vi "Cluster_Analysis.vi"(2 "Shift In":T1[](array[typedef])) -> (0 "Shift Out":T1[](array[typedef]))   [LabVIEW 2014]
uses:
  Controls/Shift_Cluster.ctl
  Controls/XY_Plot_Cluster.ctl
  Controls/Inst_type.ctl
  Globals/Meas_global.vi
  Globals/LDA_meas_global_1.vi
  Globals/LDA_meas_global_2.vi
  <vilib>/Analysis/NI_AALBase.lvlib
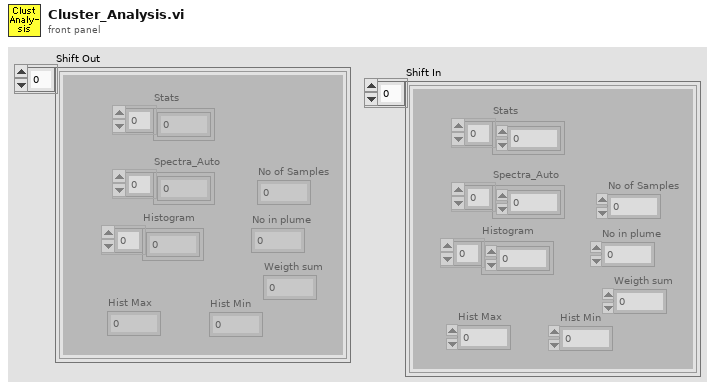
[diagram p1: front panel]
types:
  T1 = typedef "Shift_Cluster.ctl" = cluster{"Stats":dbl[], "Spectra_Auto":dbl[], "Histogram":dbl[], "Hist Max":dbl, "Hist Min":dbl, "No of Samples":i32, "No in plume":i32, "Weigth sum":dbl}
  T2 = typedef "Analysis_info_cluster.ctl" = cluster{"Colour":u32, "Inst type":T3, "Inst name":string, "Symbol":string, "Code name":string, "Extra Info":string, "Inst Array":T4, "Extra Titles":string[], "Extra Values":string[], "U":dbl, "u^2":dbl, "u^3":dbl, "u^4":dbl, "Skew_u":dbl, "Kurt_u":dbl, "Sd Error in Mean":dbl, "% u'/U":dbl, "X":dbl, "Y":dbl, "Z":dbl, "Timescale integral to 25%":dbl, "Sd Error in Variance":dbl, "Calib File":path, "Calib Constants":dbl[], "Output Position":bool, "Full Stats":bool, "Av Sampling Rate":dbl, "Av No of Samples":dbl, "Total Meas Time (s)":dbl, "ADAM Ch Name":string}
  T3 = typedef "Inst_type.ctl" = enum16{"Propeller anemometer", "Raw voltage", "Pressure Transducer", "Pitot-static tube", "Preston tube", "Hot wire", "Cross wire 1", "Cross wire 2", "Generic Linear", "Generic Polynomial", "Generic BackPoly", "Fast FID", "Thermocouple", "Cold wire", "Pulsed Wire", "LDA Vel", "LDA Tran time", "LDA Arr time", "Microphone"}
  T4 = typedef "Instrument_Array.ctl" = enum16{"PWA", "LDA", "Analogue"}
  T5 = typedef "Time_Trace_Cluster.ctl" = cluster{"Weighting":dbl[], "Time (s)":dbl[], "Voltage":dbl[], "Eng Values":dbl[]}
  T6 = typedef "XY_Plot_Cluster.ctl" = cluster{"First Name":string, "Second Name":string, "X axis name":string, "Y axis name":string, "X array":dbl[], "Y array":dbl[]}
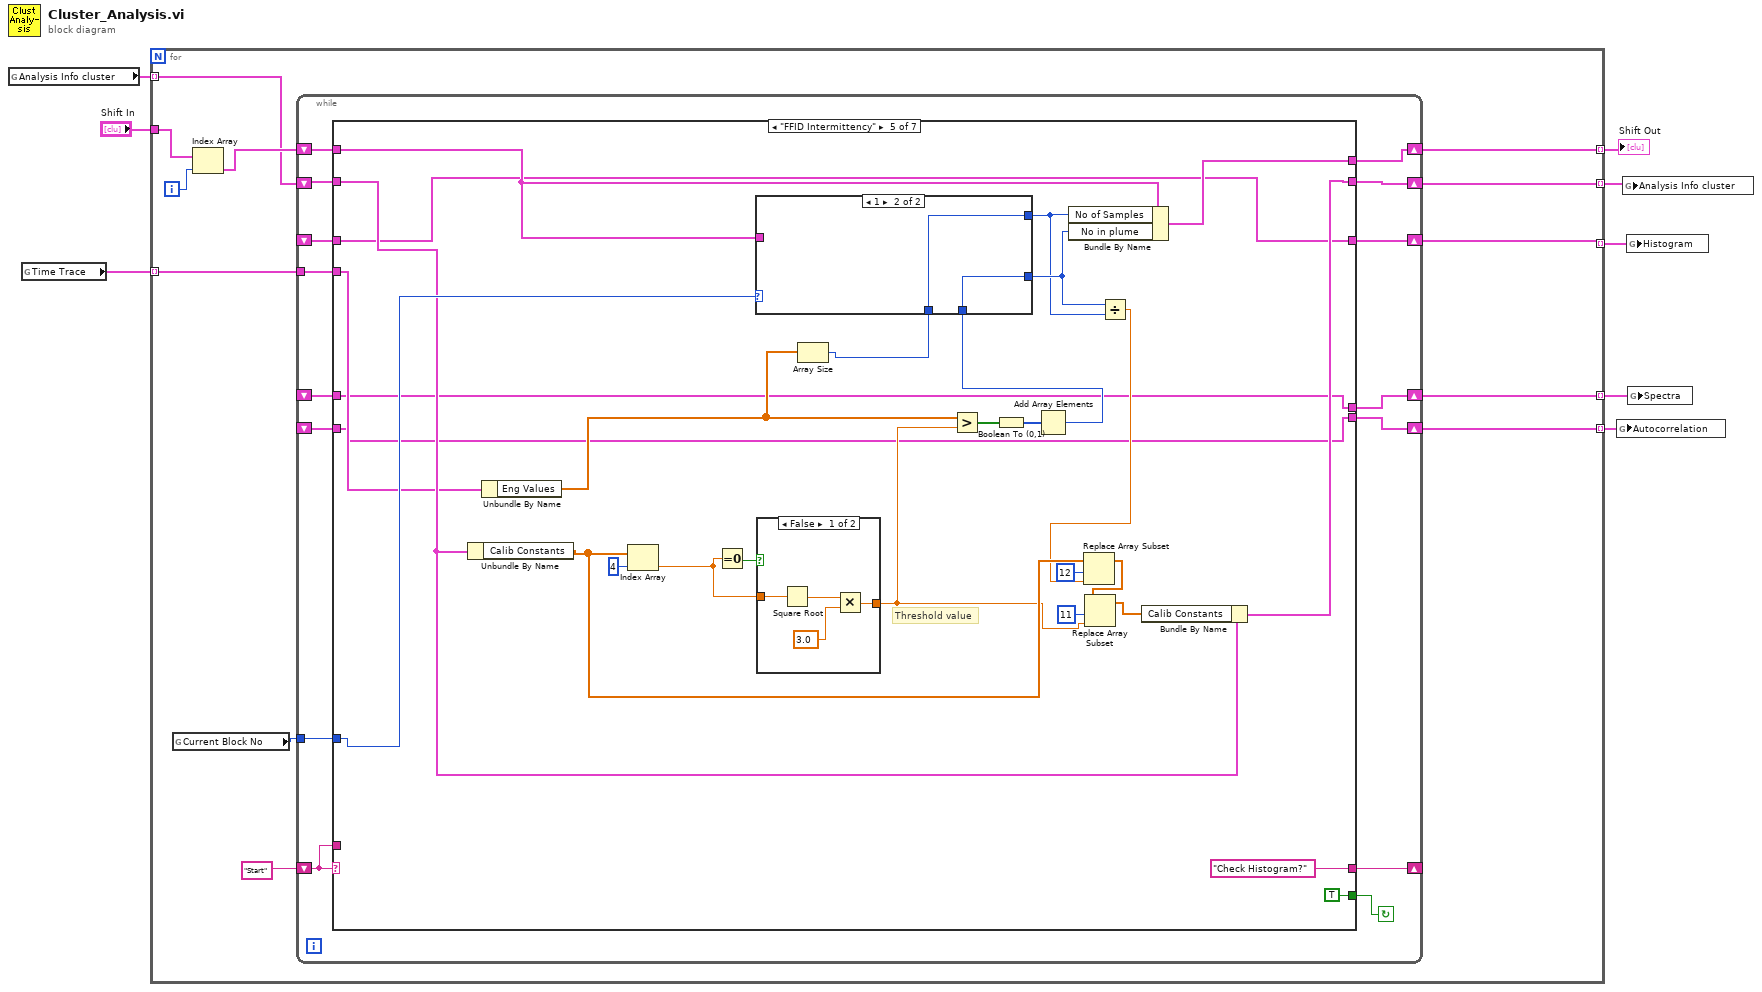
[diagram p0: block diagram]
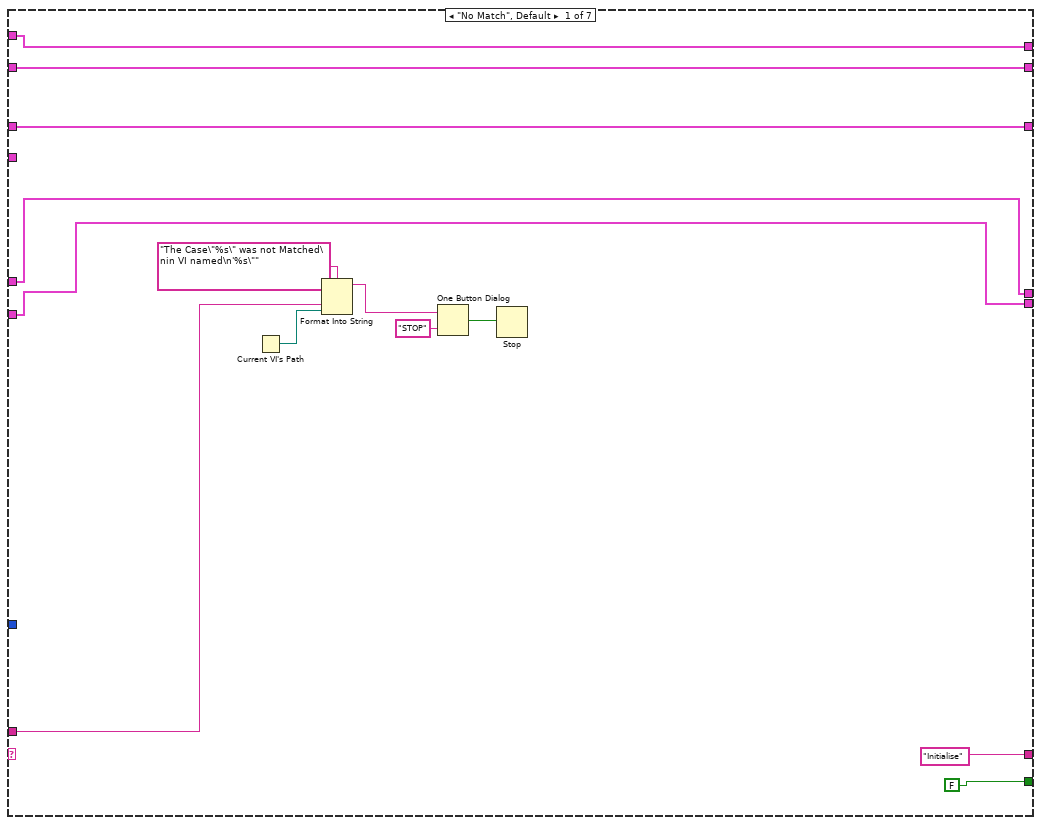
[diagram p2: hidden frame]
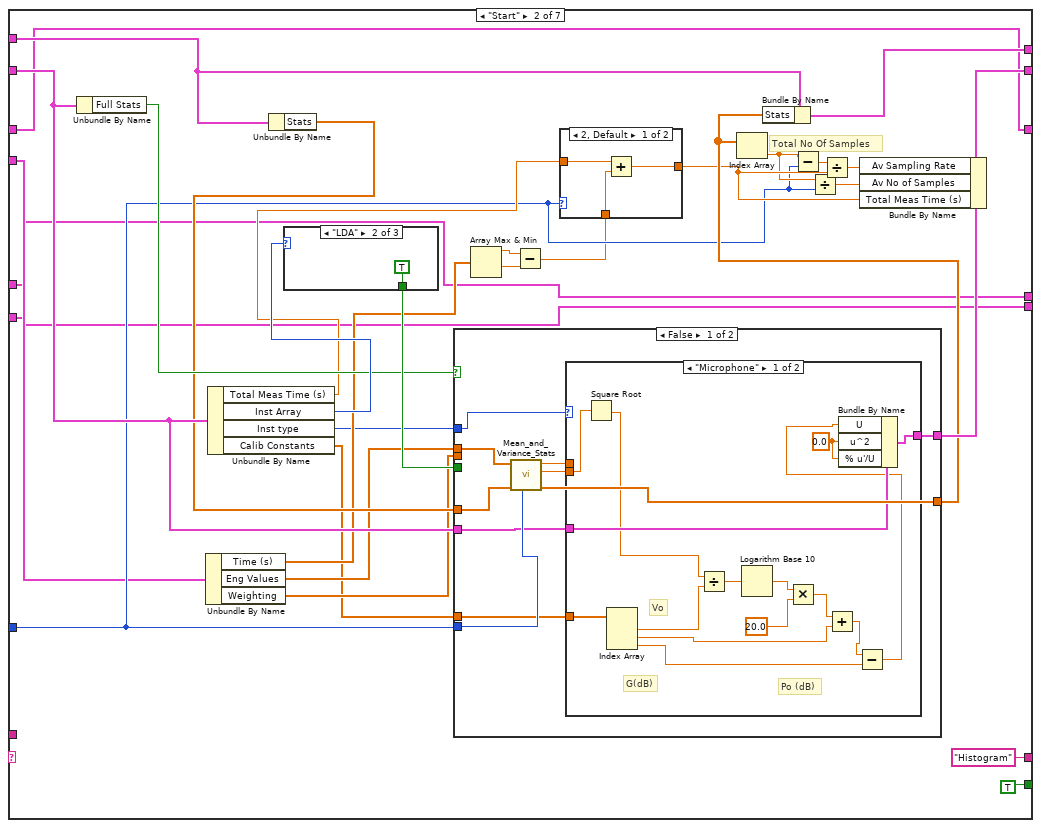
[diagram p3: hidden frame]
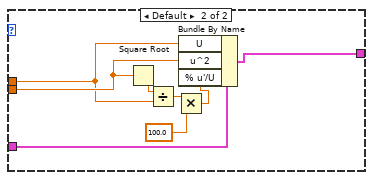
[diagram p5: hidden frame]
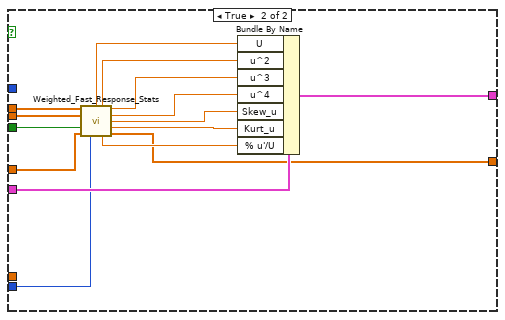
[diagram p6: hidden frame]
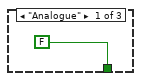
[diagram p7: hidden frame]
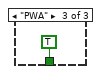
[diagram p8: hidden frame]
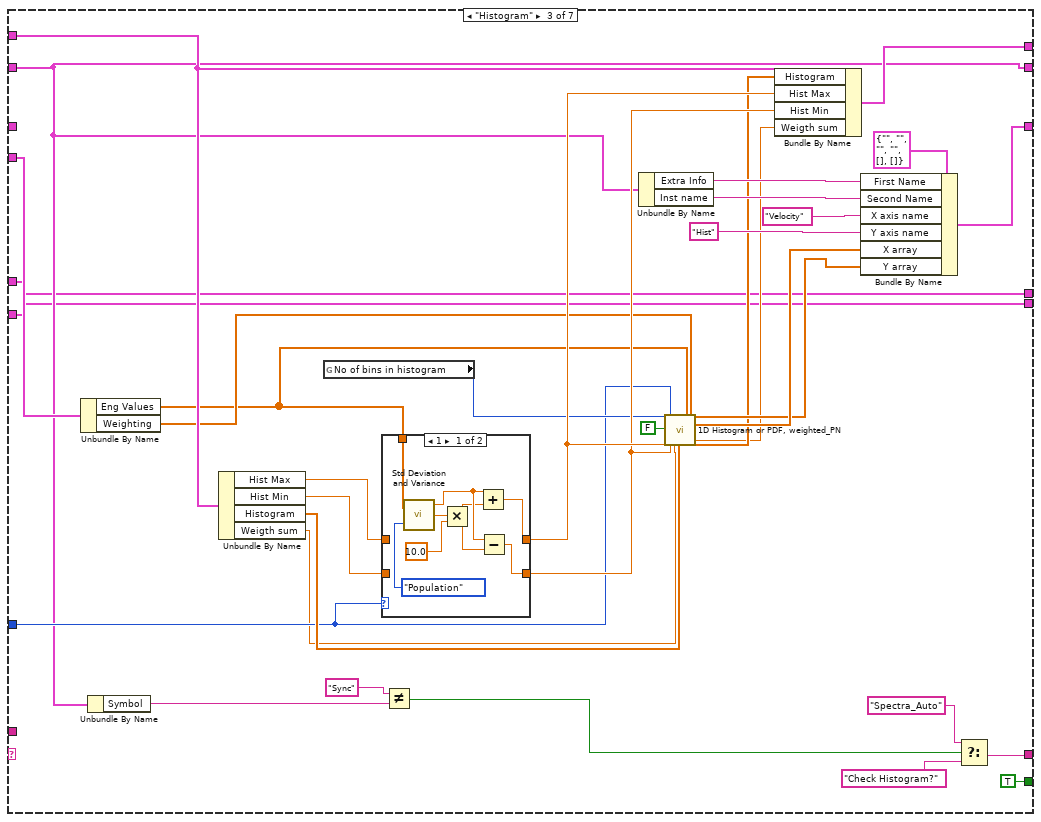
[diagram p9: hidden frame]
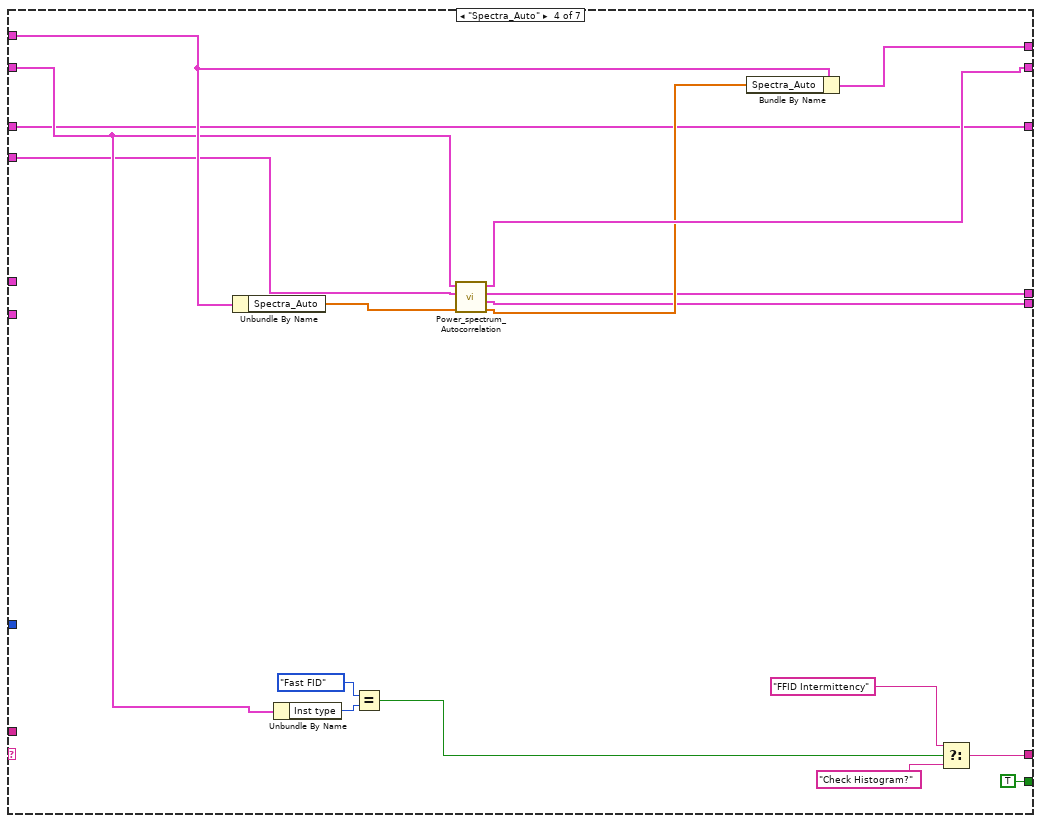
[diagram p11: hidden frame]
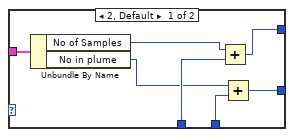
[diagram p12: hidden frame]
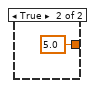
[diagram p13: hidden frame]
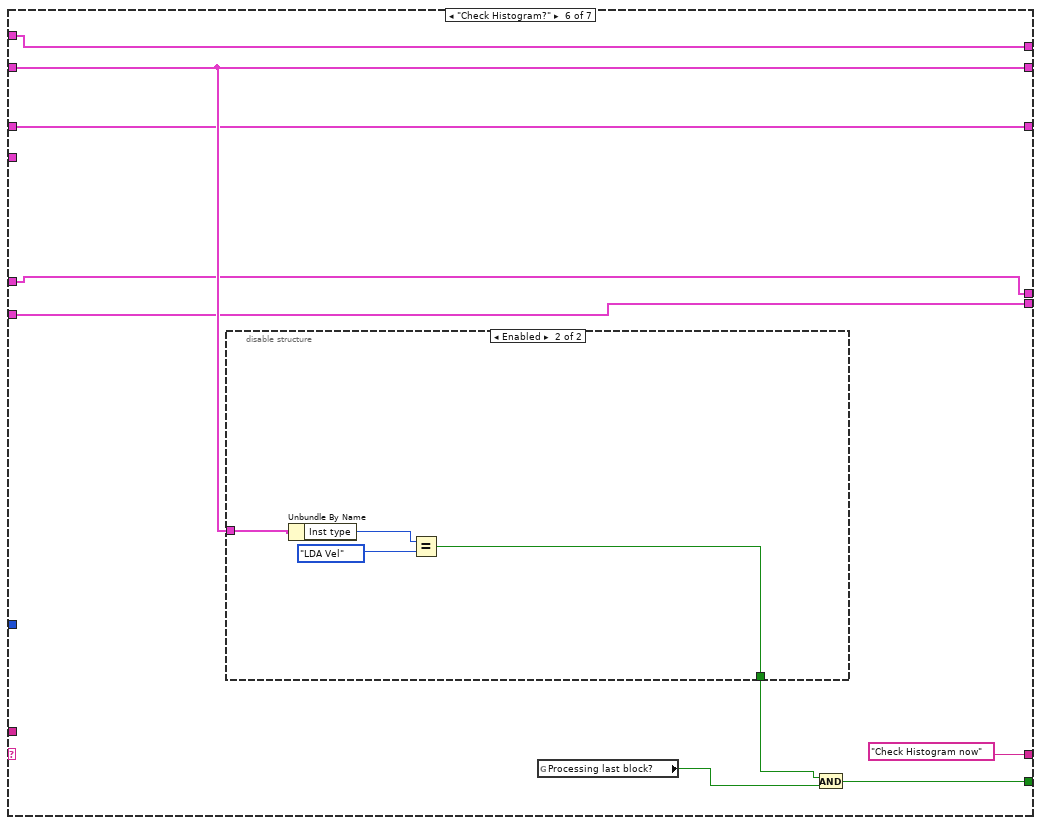
[diagram p14: hidden frame]
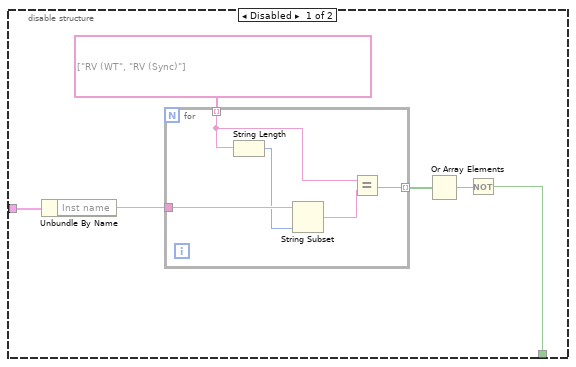
[diagram p15: hidden frame]
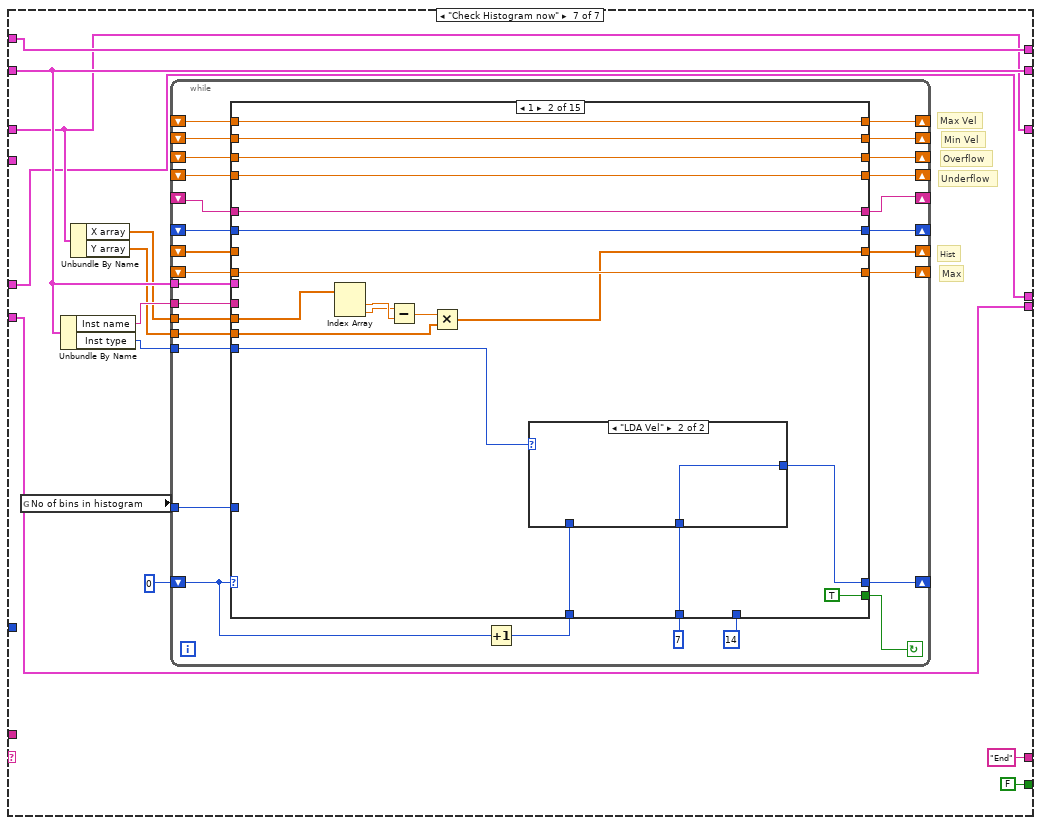
[diagram p16: hidden frame]
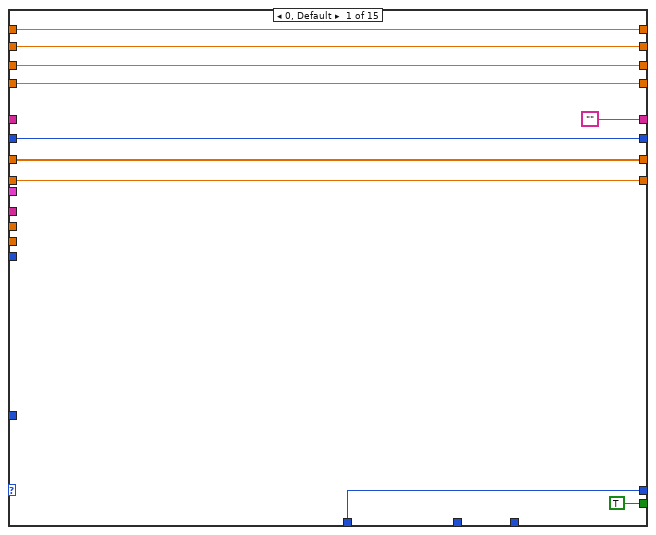
[diagram p17: hidden frame]
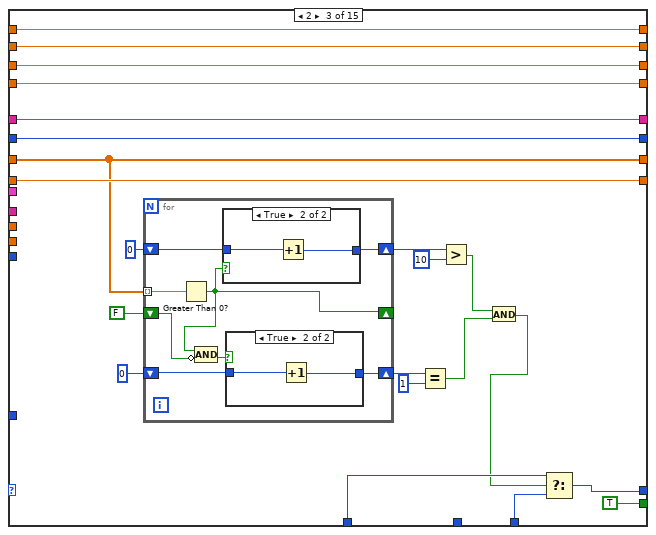
[diagram p19: hidden frame]
diagram:
  n1 = global read "Meas_global.vi" "Analysis Info cluster"() -> (w8:T2[])
  n2 = global read "Meas_global.vi" "Time Trace"() -> (w4:T5[])
  n3 = for {
    tunnel: "Shift In" -> [w18]
    tunnel: w8 -> [w16] mode=indexing
    tunnel: [w15] -> w6 mode=indexing
    tunnel: [w13] -> w5 mode=indexing
    tunnel: w4 -> [w14] mode=indexing
    tunnel: [w12] -> w3 mode=indexing
    tunnel: [w10] -> w1 mode=indexing
    tunnel: [w9] -> w2 mode=indexing
    i -> [w11]
    n4 = global read "Meas_global.vi" "Current Block No"() -> (w19:i32)
    n5 = Index Array(array=w18, index=w11) -> (element=w17:T1)
    n6 = while {
      shift-left: "Start" -> [w33]
      shift-right: [w34] -> _
      shift-right: [w31] -> w13
      shift-left: w16 -> [w32]
      shift-right: [w29] -> w15
      shift-left: w17 -> [w30]
      tunnel: w19 -> [w28]
      tunnel: w14 -> [w27]
      shift-right: [w25] -> w12
      shift-left: _ -> [w26]
      shift-right: [w24] -> w10
      shift-left: _ -> [w22]
      shift-right: [w23] -> w9
      shift-left: _ -> [w21]
      stop <- w35 continue-if-true
      n7 = case shown="\"FFID Intermittency\"" w33 {
        tunnel: [FALSE TRUE TRUE ("Processing last block?") TRUE ("Processing last block?") TRUE ("Full Stats") w242 FALSE ("Processing last block?")] -> w35
        tunnel: ["Initialise" "Histogram" w158 w184 "Check Histogram?" "Check Histogram now" ("f") "End" ("f")] -> w34
        tunnel: w33 -> [w44 _ _ _ _ _ _]
        tunnel: w32 -> [w40 w76 w137 w190 w210 w245 w267]
        tunnel: [w40 w67 w137 w193 w209 w245 w267] -> w31
        tunnel: w30 -> [w39 w73 w168 w195 w223 w246 w274]
        tunnel: [w39 w71 w167 w194 w222 w246 w274] -> w29
        tunnel: w28 -> [_ w59 w145 _ w215 _ _]
        tunnel: w27 -> [_ w58 w142 w181 w200 _ _]
        tunnel: w26 -> [w38 w54 _ w182 w198 w240 w266]
        tunnel: [w38 w54 w139 w182 w198 w240 w266] -> w25
        tunnel: [w37 w52 w136 w180 w197 w239 w263] -> w24
        tunnel: [w36 w53 w135 w179 w196 w238 w262] -> w23
        tunnel: w22 -> [w37 w52 w136 _ w197 w239 w263]
        tunnel: w21 -> [w36 w53 w135 _ w196 w238 w262]
        frame "No Match", Default {
          n8 = Current VI's Path() -> (path=w43:path)
          n9 = Format Into String(format string="The Case\"%s\" was not Matched\nin VI named\n'%s\"" ("Format String"), w44, w43) -> (resulting string=w47:string)  [unwired: 2 in, 1 out]
          n10 = One Button Dialog(message=w47, button name ("OK")="STOP") -> (true=w45:bool)
          n11 = Stop(stop? (T)=w45) -> ()
        }
        frame "Start" {
          # "Total No Of Samples"
          n12 = Unbundle By Name(w76) -> ("Full Stats"=w75:bool)
          n13 = Unbundle By Name(w58) -> ("Time (s)"=w57:dbl[], "Eng Values"=w56:dbl[], "Weighting"=w55:dbl[])
          n14 = Unbundle By Name(w76) -> ("Total Meas Time (s)"=w66:dbl, "Inst Array"=w78:T4, "Inst type"=w50:T3, "Calib Constants"=w49:dbl[])
          n15 = Unbundle By Name(w73) -> ("Stats"=w72:dbl[])
          n16 = case shown="\"LDA\"" w78 {
            tunnel: [FALSE TRUE TRUE] -> w77
            frame "Analogue" {
            }
            frame "LDA" {
            }
            frame "PWA" {
            }
          }
          n17 = case shown="False" w75 {
            tunnel: w55 -> [_ w124]
            tunnel: w56 -> [w93 w123]
            tunnel: w77 -> [_ w122]
            tunnel: w76 -> [w91 w121]
            tunnel: w72 -> [w89 w120]
            tunnel: [w88 w119] -> w65
            tunnel: [w90 w118] -> w68
            tunnel: w59 -> [w92 w117]
            tunnel: w50 -> [w85 _]
            tunnel: w49 -> [w84 _]
            frame False {
              n18 = call "Mean_and_Variance_Stats.vi"("Block No"=w92, "Shift in"=w89, "U"=w93) -> ("Shift out"=w88:dbl[], "u^2"=w87:dbl, "U"=w86:dbl)  [unwired: 3 in]
              n19 = case shown="\"Microphone\"" w85 {
                tunnel: w91 -> [w108 w116]
                tunnel: [w107 w115] -> w90
                tunnel: w87 -> [w106 w114]
                tunnel: w86 -> [_ w112]
                tunnel: w84 -> [w96 _]
                frame "Microphone" {
                  w105 = 0.0 ("u^2")
                  # "Po (dB)"
                  # "G(dB)"
                  # "Vo"
                  n20 = Square Root(x=w106) -> (sqrt(x)=w95:dbl)
                  n21 = Index Array(array=w96) -> (element #1=w97:dbl, element #2=w102:dbl, element #3=w104:dbl)  [unwired: 3 in]
                  n22 = Divide(x=w95, y=w97) -> (x/y=w98:dbl)
                  n23 = Logarithm Base 10(1:w98) -> (0:w99:dbl)
                  n24 = Multiply(x=w99, y=20.0) -> (x*y=w101:dbl)
                  n25 = Add(x=w101, y=w102) -> (x+y=w103:dbl)
                  n26 = Subtract(x=w103, y=w104) -> (x-y=w94:dbl)
                  n27 = Bundle By Name(cluster=w108, "U"=w94, "u^2"=w105, "% u'/U"=w105) -> (w107:T2)
                }
                frame Default {
                  n28 = Square Root(x=w114) -> (sqrt(x)=w113:dbl)
                  n29 = Divide(x=w113, y=w112) -> (x/y=w111:dbl)
                  n30 = Multiply(x=w111, y=100.0) -> (x*y=w109:dbl)
                  n31 = Bundle By Name(cluster=w116, "U"=w112, "u^2"=w114, "% u'/U"=w109) -> (w115:T2)
                }
              }
            }
            frame True {
              n32 = call "Weighted_Fast_Response_Stats.vi"("U"=w123, "Weighting"=w124, "Use Weighting?"=w122, "Shift in"=w120, "Block No"=w117) -> ("U"=w125:dbl, "u^2"=w126:dbl, "u^3"=w127:dbl, "u^4"=w128:dbl, "Skew"=w129:dbl, "Kurt"=w130:dbl, "% u'/U"=w131:dbl, "Shift out"=w119:dbl[])  [unwired: 3 in]
              n33 = Bundle By Name(cluster=w121, "U"=w125, "u^2"=w126, "u^3"=w127, "u^4"=w128, "Skew_u"=w129, "Kurt_u"=w130, "% u'/U"=w131) -> (w118:T2)
            }
          }
          n34 = Array Max & Min(array=w57) -> (max value=w70:dbl, min value=w69:dbl)  [unwired: 2 out]
          n35 = Subtract(x=w70, y=w69) -> (x-y=w51:dbl)
          n36 = case shown="2, Default" w59 {
            tunnel: w51 -> [w82 w83]
            tunnel: w66 -> [w81 _]
            tunnel: [w80 w83] -> w63
            frame 2, Default {
              n37 = Add(x=w81, y=w82) -> (x+y=w80:dbl)
            }
            frame 1 {
            }
          }
          n38 = Index Array(array=w65) -> (element=w61:dbl)  [unwired: 1 in]
          n39 = Bundle By Name(cluster=w73, "Stats"=w65) -> (w71:T1)
          n40 = Subtract(x=w61, y=w59) -> (x-y=w60:dbl)
          n41 = Divide(x=w61, y=w59) -> (x/y=w62:dbl)
          n42 = Divide(x=w60, y=w63) -> (x/y=w64:dbl)
          n43 = Bundle By Name(cluster=w68, "Av Sampling Rate"=w64, "Av No of Samples"=w62, "Total Meas Time (s)"=w63) -> (w67:T2)
        }
        frame "Histogram" {
          n44 = Unbundle By Name(w142) -> ("Eng Values"=w140:dbl[], "Weighting"=w141:dbl[])
          n45 = Unbundle By Name(w137) -> ("Symbol"=w155:string)
          n46 = Unbundle By Name(w168) -> ("Hist Max"=w166:dbl, "Hist Min"=w165:dbl, "Histogram"=w153:dbl[], "Weigth sum"=w144:dbl)
          n47 = global read "Meas_global.vi" "No of bins in histogram"() -> (w146:i32)
          n48 = case shown="1" w145 {
            tunnel: [w171 w178] -> w152
            tunnel: [w170 w177] -> w151
            tunnel: w140 -> [w176 _]
            tunnel: w166 -> [_ w178]
            tunnel: w165 -> [_ w177]
            frame 1 {
              n49 = call <vilib>:"Std Deviation and Variance.vi"("X"=w176, "Weighting (Sample)"=enum16{"Sample", "Population"}."Population") -> ("mean"=w175:dbl, "standard deviation"=w174:dbl)  [unwired: 1 out]
              n50 = Multiply(x=w174, y=10.0) -> (x*y=w172:dbl)
              n51 = Add(x=w175, y=w172) -> (x+y=w171:dbl)
              n52 = Subtract(x=w175, y=w172) -> (x-y=w170:dbl)
            }
            frame 2, Default {
            }
          }
          n53 = Not Equal?(x="Sync", y=w155) -> (x != y?=w154:bool)
          n54 = Unbundle By Name(w137) -> ("Extra Info"=w162:string, "Inst name"=w161:string)
          n55 = call "1D Histogram or PDF, weighted_PN.vi"("Nbins"=w146, "Mean shift"=FALSE, "max"=w152, "Current block no."=w145, "min"=w151, "Shift SumW in"=w144, "Shift PDF in"=w153, "1D data"=w140, "Weights"=w141) -> ("1D histogram or PDF"=w149:dbl[], "bin centre vals."=w150:dbl[], "Shift SumW out"=w143:dbl, "Shift PDF out"=w148:dbl[])  [unwired: 14 in, 1 out]
          n56 = Bundle By Name(cluster=w168, "Histogram"=w148, "Hist Max"=w152, "Hist Min"=w151, "Weigth sum"=w143) -> (w167:T1)
          n57 = Bundle By Name(cluster=T6 {"First Name"="", "Second Name"="", "X axis name"="", "Y axis name"="", "X array"=[], "Y array"=[]} ("element"), "First Name"=w162, "Second Name"=w161, "X axis name"="Velocity", "Y axis name"="Hist", "X array"=w150, "Y array"=w149) -> (w139:T6)
          n58 = Select(t="Spectra_Auto", s=w154, f="Check Histogram?") -> (s? t:f=w158:string)
        }
        frame "Spectra_Auto" {
          n59 = Unbundle By Name(w195) -> ("Spectra_Auto"=w192:dbl[])
          n60 = Unbundle By Name(w190) -> ("Inst type"=w189:T3)
          n61 = Equal?(x=Inst_type."Fast FID" ("Inst type"), y=w189) -> (x = y?=w187:bool)
          n62 = call "Power_spectrum_Autocorrelation.vi"("Spectrum input array"=w192, "Time Trace"=w181, "Cluster in"=w190) -> ("Spectrum output array"=w191:dbl[], "Autocorrelation"=w179:T6, "Spectra"=w180:T6, "Cluster Out"=w193:T2)  [unwired: 2 in]
          n63 = Bundle By Name(cluster=w195, "Spectra_Auto"=w191) -> (w194:T1)
          n64 = Select(t="FFID Intermittency", s=w187, f="Check Histogram?") -> (s? t:f=w184:string)
        }
        frame "FFID Intermittency" {
          # "Threshold value"
          n65 = Unbundle By Name(w210) -> ("Calib Constants"=w208:dbl[])
          n66 = Unbundle By Name(w200) -> ("Eng Values"=w199:dbl[])
          n67 = Index Array(array=w208, index=4 ("Index")) -> (element=w218:dbl)
          n68 = Equal To 0?(x=w218) -> (x = 0?=w219:bool)
          n69 = case shown="False" w219 {
            tunnel: [w234 5.0] -> w203
            tunnel: w218 -> [w233 _]
            frame False {
              n70 = Square Root(x=w233) -> (sqrt(x)=w236:dbl)
              n71 = Multiply(x=w236, y=3.0) -> (x*y=w234:dbl)
            }
            frame True {
            }
          }
          n72 = Array Size(array=w199) -> (size(s)=w214:i32)
          n73 = Greater?(x=w199, y=w203) -> (0:w216:bool[])
          n74 = Boolean To (0,1)(Boolean=w216) -> (0, 1=w217:i16[])
          n75 = Add Array Elements(numeric array=w217) -> (sum=w213:i16)
          n76 = case shown="1" w215 {
            tunnel: w223 -> [w230 _]
            tunnel: w214 -> [w228 w231]
            tunnel: w213 -> [w227 w232]
            tunnel: [w226 w232] -> w212
            tunnel: [w225 w231] -> w211
            frame 2, Default {
              n77 = Unbundle By Name(w230) -> ("No of Samples"=w229:i32, "No in plume"=w224:i32)
              n78 = Add(x=w229, y=w228) -> (x+y=w225:i32)
              n79 = Add(x=w224, y=w227) -> (x+y=w226:i32)
            }
            frame 1 {
            }
          }
          n80 = Bundle By Name(cluster=w223, "No of Samples"=w211, "No in plume"=w212) -> (w222:T1)
          n81 = Divide(x=w212, y=w211) -> (x/y=w207:dbl)
          n82 = Replace Array Subset(array=w208, new element=w207, index=12) -> (w204:dbl[])
          n83 = Replace Array Subset(array=w204, new element=w203, index=11) -> (w202:dbl[])
          n84 = Bundle By Name(cluster=w210, "Calib Constants"=w202) -> (w209:T2)
        }
        frame "Check Histogram?" {
          n85 = disable-structure shown="Enabled" {
            disable-tunnel: w245 -> [w252 w261]
            disable-tunnel: [w247 w258] -> w241
            frame Disabled {
              n86 = Unbundle By Name(w252) -> ("Inst name"=w250:string)
              n87 = for {
                tunnel: string[] ["RV (WT", "RV (Sync)"] ("appended array") -> [w254] mode=indexing
                tunnel: w250 -> [w257]
                tunnel: [w253] -> w249 mode=indexing
                n88 = String Length(string=w254) -> (length=w256:i32)
                n89 = String Subset(string=w257, length (rest)=w256) -> (substring=w255:string)  [unwired: 1 in]
                n90 = Equal?(x=w254, y=w255) -> (x = y?=w253:bool)
              }
              n91 = Or Array Elements(Boolean array=w249) -> (logical OR=w248:bool)
              n92 = Not(x=w248) -> (.not. x?=w247:bool)
            }
            frame Enabled {
              n93 = Unbundle By Name(w261) -> ("Inst type"=w259:T3)
              n94 = Equal?(x=w259, y=Inst_type."LDA Vel" ("Inst type")) -> (x = y?=w258:bool)
            }
          }
          n95 = global read "Meas_global.vi" "Processing last block?"() -> (w243:bool)
          n96 = And(x=w241, y=w243) -> (x .and. y?=w242:bool)
        }
        frame "Check Histogram now" {
          # "Underflow"
          # "Overflow"
          # "Min Vel"
          # "Max Vel"
          # "Max"
          # "Hist"
          n97 = global read "Meas_global.vi" "No of bins in histogram"() -> (w271:i32)
          n98 = Unbundle By Name(w267) -> ("Inst name"=w268:string, "Inst type"=w269:T3)
          n99 = Unbundle By Name(w266) -> ("X array"=w265:dbl[], "Y array"=w264:dbl[])
          n100 = while {
            tunnel: w271 -> [w290]
            shift-left: _ -> [w291]
            shift-right: [w293] -> _
            shift-left: _ -> [w292]
            shift-right: [w294] -> _
            shift-left: _ -> [w295]
            shift-right: [w296] -> _
            shift-left: _ -> [w297]
            shift-right: [w298] -> _
            shift-left: 0 -> [w301]
            shift-right: [w299] -> _
            shift-right: [w287] -> _
            shift-left: _ -> [w285]
            shift-right: [w286] -> _
            shift-left: _ -> [w284]
            shift-right: [w283] -> _
            shift-left: _ -> [w280]
            shift-right: [w282] -> _
            shift-left: _ -> [w281]
            tunnel: w269 -> [w279]
            tunnel: w265 -> [w278]
            tunnel: w264 -> [w277]
            tunnel: w268 -> [w276]
            tunnel: w267 -> [w275]
            stop <- w302 continue-if-true
            n101 = Increment(x=w301) -> (x+1=w300:i32)
            n102 = case shown="1" w301 {
              tunnel: [TRUE TRUE TRUE TRUE TRUE TRUE TRUE TRUE TRUE TRUE TRUE TRUE TRUE TRUE FALSE] -> w302
              tunnel: w300 -> [w312 w326 w340 w385 w416 w431 _ w476 w501 w536 w561 w582 w589 w610 w612]
              tunnel: [w312 w327 w338 w387 w416 w439 w465 w476 w501 w536 w563 w582 w591 w610 w612] -> w299
              tunnel: [w307 w329 w353 w373 w408 w422 w460 w478 w508 w543 w564 w578 w592 w606 w614] -> w298
              tunnel: w297 -> [w307 w329 w353 _ w408 _ w460 w478 w508 w543 w564 w578 w592 w606 w614]
              tunnel: ["" w328 w352 w386 w414 w438 w467 w480 w509 w544 w567 w580 w595 w608 w615] -> w296
              tunnel: w295 -> [_ w328 w352 w386 w415 w438 w468 w480 w509 w544 w567 w581 w595 w609 w615]
              tunnel: [w310 w313 w350 w378 w412 w428 w466 w479 w504 w539 w566 w579 w594 w607 w623] -> w294
              tunnel: [w309 w320 w351 w376 w411 w426 w462 w477 w502 w537 w565 w574 w593 w602 w622] -> w293
              tunnel: w292 -> [w310 _ w350 w378 w412 w428 w466 w479 w504 w539 w566 w579 w594 w607 w623]
              tunnel: w291 -> [w309 w320 w351 _ w411 _ w462 _ w502 w537 w565 w574 w593 w602 w622]
              tunnel: w290 -> [_ _ _ w379 _ w435 _ _ w490 w524 _ _ _ _ _]
              tunnel: 7 -> [_ w325 _ _ _ _ _ _ _ _ _ _ _ _ _]
              tunnel: 14 ("y") -> [_ _ w339 _ _ w430 w465 _ _ _ _ _ _ _ _]
              tunnel: [w306 w324 w336 w372 w406 w421 w458 w474 w496 w532 w559 w570 w587 w601 w621] -> w287
              tunnel: [w305 w323 w335 w371 w405 w420 w457 w473 w497 w531 w558 w573 w586 w598 w620] -> w286
              tunnel: w285 -> [w306 w324 w336 w372 w406 w421 w458 _ w496 w532 w559 w570 w587 w601 w621]
              tunnel: w284 -> [w305 w323 w335 w371 w405 w420 w457 _ w497 w531 w558 w573 w586 w598 w620]
              tunnel: [w303 w321 w333 w369 w403 w418 w455 w471 w495 w530 w556 w571 w585 w600 w618] -> w283
              tunnel: [w304 w322 w334 w370 w404 w419 w456 w472 w494 w529 w557 w572 w584 w599 w619] -> w282
              tunnel: w281 -> [w304 w322 w334 w370 w404 w419 w456 w472 w494 _ w557 w572 w584 w599 w619]
              tunnel: w280 -> [w303 w321 w333 w369 w403 w418 w455 w471 _ w530 w556 w571 w585 w600 w618]
              tunnel: w279 -> [_ w319 _ _ _ _ _ _ _ _ _ _ _ _ _]
              tunnel: w278 -> [_ w316 _ _ w401 _ w453 _ w486 w521 _ _ _ _ _]
              tunnel: w277 -> [_ w314 _ _ _ _ _ _ _ _ _ _ _ _ _]
              tunnel: w276 -> [_ _ _ _ w402 _ w454 _ _ _ _ w569 _ w597 _]
              tunnel: w275 -> [_ _ _ _ _ _ _ w470 _ _ _ _ _ _ _]
              frame 0, Default {
              }
              frame 1 {
                n103 = Index Array(array=w316) -> (element #1=w318:dbl, element #2=w317:dbl)  [unwired: 2 in]
                n104 = Subtract(x=w317, y=w318) -> (x-y=w315:dbl)
                n105 = Multiply(x=w315, y=w314) -> (x*y=w313:dbl[])
                n106 = case shown="\"LDA Vel\"" w319 {
                  tunnel: [w331 w332] -> w327
                  tunnel: w326 -> [w331 _]
                  tunnel: w325 -> [_ w332]
                  frame "Propeller anemometer", Default {
                  }
                  frame "LDA Vel" {
                  }
                }
              }
              frame 2 {
                n107 = for {
                  tunnel: w350 -> [w362] mode=indexing
                  shift-right: [w355] -> _
                  shift-left: FALSE -> [w361]
                  shift-right: [w358] -> w344
                  shift-left: 0 -> [w359]
                  shift-right: [w356] -> w346
                  shift-left: 0 -> [w357]
                  n108 = Greater Than 0?(x=w362) -> (x > 0?=w355:bool)
                  n109 = Compound Arithmetic op=AND(w355, invert w361) -> (w360:bool)
                  n110 = case shown="True" w355 {
                    tunnel: w357 -> [w363 w365]
                    tunnel: [w363 w364] -> w356
                    frame False {
                    }
                    frame True {
                      n111 = Increment(x=w365) -> (x+1=w364:i32)
                    }
                  }
                  n112 = case shown="True" w360 {
                    tunnel: w359 -> [w366 w368]
                    tunnel: [w366 w367] -> w358
                    frame False {
                    }
                    frame True {
                      n113 = Increment(x=w368) -> (x+1=w367:i32)
                    }
                  }
                }
                n114 = Equal?(x=w344, y=1) -> (x = y?=w341:bool)
                n115 = Greater?(x=w346, y=10) -> (0:w342:bool)
                n116 = And(x=w342, y=w341) -> (x .and. y?=w337:bool)
                n117 = Select(t=w340, s=w337, f=w339) -> (s? t:f=w338:i32)
              }
              frame 3 {
                # "Clipping?"
                n118 = Increment(x=w379) -> (x+1=w392:i32)
                n119 = while {
                  tunnel: [w393] -> w376
                  tunnel: w378 -> [w400]
                  shift-left: 0.0 -> [w393]
                  shift-right: [w398] -> w389
                  shift-left: w392 -> [w399]
                  shift-right: [w397] -> w375
                  stop <- w394 continue-if-true
                  n120 = Decrement(x=w399) -> (x-1=w397:i32)
                  n121 = Index Array(array=w400, index=w399) -> (element=w398:dbl)
                  n122 = Equal To 0?(x=w393) -> (x = 0?=w395:bool)
                  n123 = Greater Than 0?(x=w397) -> (x > 0?=w396:bool)
                  n124 = And(x=w396, y=w395) -> (x .and. y?=w394:bool)
                }
                n125 = Greater?(x=w376, y=0.04) -> (0:w381:bool)
                n126 = Multiply(x=w376, y=0.7) -> (x*y=w390:dbl)
                n127 = Add(x=w375, y=2) -> (x+y=w373:i32)
                n128 = Increment(x=w385) -> (x+1=w384:i32)
                n129 = Greater?(x=w390, y=w389) -> (0:w382:bool)
                n130 = And(x=w381, y=w382) -> (x .and. y?=w380:bool)
                n131 = Select(t=w385, s=w380, f=w384) -> (s? t:f=w387:i32)
              }
              frame 4 {
                n132 = Index Array(array=w401, index=w408) -> (element=w407:dbl)
                n133 = Multiply(x=w411, y=100.0) -> (x*y=w409:dbl)
                n134 = Format Into String(format string="Histogram of %s may indicate Clipping at Upper limit of %.2f by %.0f%%.\\n" ("Format String"), initial string=w415, w402, w407, w409) -> (resulting string=w414:string)  [unwired: 1 in, 1 out]
              }
              frame 5 {
                # "Clipping?"
                n135 = Array Max & Min(array=w428) -> (max value=w427:dbl)  [unwired: 3 out]
                n136 = while {
                  tunnel: w435 -> [w445]
                  tunnel: [w447] -> w426
                  tunnel: w428 -> [w452]
                  shift-left: 0.0 -> [w447]
                  shift-right: [w450] -> w441
                  shift-left: 0 -> [w451]
                  shift-right: [w446] -> w424
                  stop <- w448 continue-if-true
                  n137 = Increment(x=w451) -> (x+1=w446:i32)
                  n138 = Index Array(array=w452, index=w451) -> (element=w450:dbl)
                  n139 = Less?(x=w446, y=w445) -> (x < y?=w444:bool)
                  n140 = Equal To 0?(x=w447) -> (x = 0?=w449:bool)
                  n141 = And(x=w444, y=w449) -> (x .and. y?=w448:bool)
                }
                n142 = Not Equal?(x=w426, y=w427) -> (x != y?=w425:bool)
                n143 = Greater?(x=w426, y=0.04) -> (0:w433:bool)
                n144 = Multiply(x=w426, y=0.45) -> (x*y=w442:dbl)
                n145 = Subtract(x=w424, y=2) -> (x-y=w422:i32)
                n146 = Greater?(x=w442, y=w441) -> (0:w434:bool)
                n147 = Compound Arithmetic op=AND(w425, w433, w434) -> (w432:bool)
                n148 = Select(t=w431, s=w432, f=w430) -> (s? t:f=w439:i32)
              }
              frame 6 {
                n149 = Index Array(array=w453, index=w460) -> (element=w459:dbl)
                n150 = Multiply(x=w462, y=100.0) -> (x*y=w461:dbl)
                n151 = Format Into String(format string="Histogram of %s may indicate Clipping at Lower limit of %.2f by %.0f%%.\\n" ("Format String"), initial string=w468, w454, w459, w461) -> (resulting string=w467:string)  [unwired: 1 in, 1 out]
              }
              frame 7 {
                n152 = Unbundle By Name(w470) -> ("Code name"=w475:string)
                n153 = case shown="\"1LDA:U\", Default" w475 {
                  tunnel: [w483 w485] -> w474
                  tunnel: [w482 w484] -> w473
                  frame "1LDA:U", Default {
                    n154 = global read "LDA_meas_global_1.vi" "Max Vel BSA1"() -> (w483:dbl)
                    n155 = global read "LDA_meas_global_1.vi" "Min Vel BSA1"() -> (w482:dbl)
                  }
                  frame "2LDA:U" {
                    n156 = global read "LDA_meas_global_2.vi" "Max Vel BSA2"() -> (w485:dbl)
                    n157 = global read "LDA_meas_global_2.vi" "Min Vel BSA2"() -> (w484:dbl)
                  }
                }
                n158 = Add Array Elements(numeric array=w479) -> (sum=w477:dbl)
              }
              frame 8 {
                n159 = Divide(x=w490, y=2) -> (x/y=w488:dbl)
                n160 = Array Max & Min(array=w486) -> (max value=w493:dbl, min value=w492:dbl)  [unwired: 2 out]
                n161 = Subtract(x=w493, y=w492) -> (x-y=w491:dbl)
                n162 = Divide(x=w491, y=w488) -> (x/y=w487:dbl)
                n163 = Subtract(x=w496, y=w487) -> (x-y=w507:dbl)
                n164 = for {
                  tunnel: w507 -> [w514]
                  shift-right: [w512] -> w503
                  shift-left: 0.0 -> [w515]
                  tunnel: w504 -> [w516] mode=indexing
                  tunnel: w486 -> [w511] mode=indexing
                  n165 = Greater?(x=w511, y=w514) -> (0:w513:bool)
                  n166 = case shown="False" w513 {
                    tunnel: w516 -> [_ w519]
                    tunnel: w515 -> [w517 w520]
                    tunnel: [w517 w518] -> w512
                    frame False {
                    }
                    frame True {
                      n167 = Add(x=w520, y=w519) -> (x+y=w518:dbl)
                    }
                  }
                }
                n168 = Divide(x=w503, y=w502) -> (x/y=w499:dbl)
                n169 = Greater?(x=w499, y=0.025) -> (0:w500:bool)
                n170 = Select(t=w499, s=w500, f=0.0) -> (s? t:f=w495:dbl)
              }
              frame 9 {
                n171 = Divide(x=w524, y=2) -> (x/y=w523:dbl)
                n172 = Array Max & Min(array=w521) -> (max value=w528:dbl, min value=w527:dbl)  [unwired: 2 out]
                n173 = Subtract(x=w528, y=w527) -> (x-y=w526:dbl)
                n174 = Divide(x=w526, y=w523) -> (x/y=w522:dbl)
                n175 = Add(x=w531, y=w522) -> (x+y=w542:dbl)
                n176 = for {
                  tunnel: w542 -> [w549]
                  shift-right: [w547] -> w538
                  shift-left: 0.0 -> [w550]
                  tunnel: w539 -> [w551] mode=indexing
                  tunnel: w521 -> [w546] mode=indexing
                  n177 = Less?(x=w546, y=w549) -> (x < y?=w548:bool)
                  n178 = case shown="True" w548 {
                    tunnel: w551 -> [_ w554]
                    tunnel: w550 -> [w552 w555]
                    tunnel: [w552 w553] -> w547
                    frame False {
                    }
                    frame True {
                      n179 = Add(x=w555, y=w554) -> (x+y=w553:dbl)
                    }
                  }
                }
                n180 = Divide(x=w538, y=w537) -> (x/y=w534:dbl)
                n181 = Greater?(x=w534, y=0.025) -> (0:w535:bool)
                n182 = Select(t=w534, s=w535, f=0.0) -> (s? t:f=w529:dbl)
              }
              frame 10 {
                n183 = Equal To 0?(x=w556) -> (x = 0?=w562:bool)
                n184 = Increment(x=w561) -> (x+1=w560:i32)
                n185 = Select(t=w560, s=w562, f=w561) -> (s? t:f=w563:i32)
              }
              frame 11 {
                n186 = Multiply(x=w571, y=100.0) -> (x*y=w575:dbl)
                n187 = Format Into String(format string="%.1f %% of the %s samples are too close to the upper velocity limit of %.2f m/s.\n" ("Format String"), initial string=w581, w575, w569, w570) -> (resulting string=w580:string)  [unwired: 1 in, 1 out]
              }
              frame 12 {
                n188 = Equal To 0?(x=w584) -> (x = 0?=w590:bool)
                n189 = Increment(x=w589) -> (x+1=w588:i32)
                n190 = Select(t=w588, s=w590, f=w589) -> (s? t:f=w591:i32)
              }
              frame 13 {
                n191 = Multiply(x=w599, y=100.0) -> (x*y=w603:dbl)
                n192 = Format Into String(format string="%.1f %% of the %s samples are too close to the lower velocity limit of %.2f m/s.\n" ("Format String"), initial string=w609, w603, w597, w598) -> (resulting string=w608:string)  [unwired: 1 in, 1 out]
              }
              frame 14 {
                n193 = global read "Meas_global.vi" "Over/Under string"() -> (w617:string)
                n194 = Concatenate Strings(w617, w615) -> (w616:string)
                n195 = global write "Meas_global.vi" "Over/Under string"(w616) -> ()
              }
            }
          }
        }
      }
    }
  }
  "Shift Out" <- w6
  n196 = global write "Meas_global.vi" "Autocorrelation"(w2) -> ()
  n197 = global write "Meas_global.vi" "Analysis Info cluster"(w5) -> ()
  n198 = global write "Meas_global.vi" "Histogram"(w3) -> ()
  n199 = global write "Meas_global.vi" "Spectra"(w1) -> ()
